vi "GUI_Bella_Control_Center_OFI.vi"() -> ()   [LabVIEW 2020]
uses:
  Shared/GUI_Template/GUI_master/tcp_new_data_event.ctl
  Shared/GUI_Template/GUI_master/tcp new data cluster.ctl
  GUI_TestStand/Fire button.ctl
  Device Drivers/DG645/subVIs/TriggerSource_TypDef.ctl
  Jet on times.ctl
  <vilib>/Utility/config.llb/Write Key (I32).vi
  <vilib>/Platform/browser.llb/Open URL in Default Browser (string).vi
  <vilib>/Utility/config.llb/NI_LVConfig.lvlib
panel:
  out "Jet On Times":T1 {"gas jet on time" format="%#_6p"}
  in  "value10::42":dbl=0.006 caption="JetOnTime H" min=0.0 max=0.01 format="%#_6p"
  in  "value9::42":dbl=0.006 caption="JetOnTime F" min=0.0 max=0.01 format="%#_6p"
  in  "value8::42":dbl=0.006 caption="JetOnTime D" min=0.0 max=0.01 format="%#_6p"
  in  "Delay.Ch H::32":dbl caption="Time width H" min=-0.1 max=0.01 format="%.3p"
  in  "Delay.Ch G::32":dbl caption="jet open G" min=-0.1 max=0.1 format="%.3p"
  in  "Delay.Ch D::32":dbl caption="Time Width D" min=-0.1 max=0.01 format="%.3p"
  in  "Delay.Ch E::32":dbl caption="jet open E" min=-0.1 max=0.03 format="%.3p"
  in  "Delay.Ch F::32":dbl caption="Time width F" min=-0.1 max=0.01 format="%.3p"
  in  "Delay.Ch C::32":dbl caption="jet open C" min=-0.1 max=0.1 format="%.3p"
  out "got manpar ofi bool data":bool
  out "got manpar ofi data":bool
  out "set expt editor":bool
  in  "Delay.Ch B::10":dbl=-1.631e-06 caption="UniblitzOpenTime\n(0 closed, 0.07 default)" min=-0.1 max=0.08 format="%.4f"
  in  "Delay.Ch D::10":dbl=-1.631e-06 caption="Delay D" min=-0.1 max=0.01 format="%.4f"
  in  "value6::42":dbl=0.006 caption="PostScanRate" min=0.1 max=1.0 format="%#_3f"
  in  "value5::42":dbl=0.006 caption="1BL-2BL-\nSplitter-Rpcnt" min=-9999999.0 max=9999999.0 format="%#_6p"
  in  "value6::43":bool=TRUE caption="GhostFoil-In"
  in  "value5::43":bool=TRUE caption="1BL-Energy\nMeter-In"
  in  "value4::43":bool=TRUE caption="2BLFoil-In"
  in  "value3::43":bool=TRUE caption="1BLFoil-In"
  in  "value2::43":bool=TRUE caption="ClunkerIn"
  out "CurrentStatus":string
  in  "MoveStage":bool
  in  "Position.Ch1::44":dbl caption="Current Position" min=0.0 max=150.0
  in  "GUIdevice 44":string="STAGE-LT-Megattenuator"
  in  "GUIdevice 43":string="MANPAR-BELLA-OFI-Boolean"
  in  "GUIdevice 42":string="MANPAR-BELLA-OFI"
  in  "Pressure.device 2::39":dbl caption="Dopant pressure\nLow1down" min=-20.0 max=500.0 format="%.3f"
  out "HPD2 to match HPD":dbl
  in  "Save \ncreenshots":bool
  out "error out":errorcluster
  out "Hpd pos for jet exit":dbl
  in  "value2::42":dbl=276.0 caption="jet exit on hpd for hexX=0" min=-9999999.0 max=9999999.0
  in  "GUIdevice 41":string="STAGE-PL1-JetLength"
  in  "position::41":dbl caption="Jet Length pos" min=0.0 max=50.0 format="%.1f"
  out "lp mode HPDplane\n - HPD ref pos":dbl
  out "height above jet":dbl
  in  "value3::42":dbl=2.6 caption="zpos for 0 above jet" min=-9999999.0 max=9999999.0
  out "HPD - focus":dbl
  in  "value1::42":dbl=230.0 caption="focus on HPD" min=-9999999.0 max=9999999.0
  out "1BL delay (ns)\n+ is 1BL after 2BL":dbl
  in  "Position.Axis 1::8":dbl caption="1BL delay (mm)" min=-500.0 max=500.0 format="%.1f"
  in  "GUIdevice 8":string="STAGE-LT-1BLDelay"
  in  "value4::42":dbl=0.006 caption="JetOnTime B" min=-9999999.0 max=9999999.0 format="%#_6p"
  in  "Position.Channel 5::25":dbl caption="SMFiber (45in, 1out)" min=-60.0 max=55.0 format="%.1f"
  in  "value1::43":bool=TRUE caption="GasJetOn"
  in  "value0::43":bool=TRUE caption="SCS"
  in  "Thales.DIAG_CU_Output_Percent_1::37":dbl caption="Amp2 att (%)" min=1.0 max=100.0 step=500.0 format="%.2f"
  in  "GUIdevice 37":string="SVE-LT-Thales"
  in  "Pressure.device 1::39":dbl caption="Hydrogen pressure\nHigh500" min=-20.0 max=500.0 format="%.3f"
  in  "GUIdevice 39":string="PRC-PL1-HighPressure"
  in  "Scan":T2(ring)
  in  "LogTable":bool
  in  "New Google\nExpLog for new day?":bool=TRUE
  out "standard output":string
  in  "Create Log":bool caption="LogTable"
  in  "GUIdevice 38":string="STAGE-2BL-Compressor"
  in  "Position.Axis 1::38":dbl caption="Comp2 Translation" min=0.0 max=20.0 format="%.3f"
  in  "Position.Channel 5::31":T3(ring) caption="FROG foil"
  in  "Position.Channel 2::31":T3(ring) caption="Little Rick"
  in  "AnalogOutput.Channel 1::36":dbl caption="M4A att (V)" min=0.0 max=5.0 step=500.0 format="%.2f"
  in  "GUIdevice 36":string="ATT-2BL-M4A"
  in  "GUIdevice 35":string="ATT-2BL-DM"
  in  "AnalogOutput.Channel 1::35":dbl caption="2BL DM att (V)" min=0.0 max=5.0 step=500.0 format="%.2f"
  in  "Step size 2":dbl=20.0 caption="Step size" min=-22.0 max=22.0
  in  "Position.Axis 4::33":dbl caption="Holy M V F4" min=-100000.0 max=100000.0 step=500.0
  in  "Position.Axis 3::33":dbl caption="Holy M H F3" min=-1000000.0 max=1000000.0 step=500.0
  in  "Position.Axis 2::33":dbl caption="Bessel M3 V F2" min=-100000.0 max=100000.0 step=500.0
  in  "Position.Axis 1::33":dbl caption="Bessel M3 H F1" min=-100000.0 max=100000.0 step=500.0
  in  "GUIdevice 33":string="MCD-PL1-picosOFI1"
  in  "Delay.Ch B::32":dbl caption="Time width B" min=-0.1 max=0.01 format="%.3p"
  in  "Delay.Ch A::32":dbl caption="jet open A" min=-0.1 max=0.1 format="%.3p"
  in  "GUIdevice 32":string="DDG-AA-SRSGasJet-645"
  in  "position::6":dbl caption="LPmode stage long (605 safe)" min=0.0 max=605.0 format="%.1f"
  in  "GUIdevice 6":string="STAGE-PL1-LPmodeLong"
  in  "EnableMotor::6":bool caption="LPmode motor \nstatus"
  in  "GUIdevice 4":string="STAGE-PL1-Capstage1"
  in  "GUIdevice 31":string="1WIRE-BELLA-Flipper"
  in  "Amplitude.Ch GH::10":dbl=-1.631e-06 caption="Shot Shutter V" min=0.5 max=5.0 format="%.1f"
  in  "Rate (Hz)":dbl=0.3
  out "Crystal2":enum16{"In", "Out", "Unknown"}(ring)
  in  "wangle::28":dbl caption="w" min=-2.0 max=2.0 step=0.01 format="%.5f"
  in  "vangle::28":dbl caption="v" min=-5.0 max=5.0 step=0.01 format="%.5f"
  in  "uangle::28":dbl caption="u" min=-1.0 max=1.0 step=0.01 format="%.5f"
  in  "ypos::28":dbl caption="y" min=-3.0 max=3.0 step=0.01 format="%.5f"
  in  "zpos::28":dbl caption="z" min=-12.5 max=12.5 step=0.01 format="%.5f"
  in  "xpos::28":dbl caption="x" min=-0.5 max=0.5 step=0.01 format="%.5f"
  in  "GUIdevice 28":string="HEX-PL1-2"
  in  "Position.Channel 1::25":dbl caption="LPmode kicker (~1in, 75out)" min=-75.0 max=79.0 format="%.1f"
  in  "GUIdevice 25":string="STAGE-PL1-Smaract"
  in  "Heater Alignment Directions":bool
  in  "Position.Axis 3::15":dbl caption="XY" min=-3.0 max=16.0 format="%.4f"
  in  "Position.Axis 2::15":dbl caption="Y" min=-3.0 max=17.0 format="%.4f"
  in  "Position.Axis 1::15":dbl caption="X" min=-3.0 max=13.0 format="%.4f"
  in  "GUIdevice 24":string="STAGE-HEAT-TL1"
  in  "Encoder position::23":dbl caption="position HPD2" min=0.0 max=600.0 format="%.1f"
  in  "position::3":dbl caption="position HPD" min=0.0 max=600.0 format="%.1f"
  in  "GUIdevice 23":string="STAGE-HPD-Far"
  in  "GUIdevice 22":string="MANPAR-BELLA-FireCont"
  in  "Allow Fire Continues":bool
  out "Fire continues Indicator":bool caption="firing"
  in  "Fire Button":T4=TRUE
  in  "Trigger.Source::10":T5 caption="SRS Trigger Mode"
  out "Absolute discharge timing":dbl caption="delay from pk" format="%#.3p"
  in  "Delay.Ch E::17":dbl caption="Timing box" min=-0.1 max=0.1 format="%.3p"
  in  "value0::22":bool caption="Fire continuosly"
  in  "GUIdevice 15":string="MCD-HEAT-ESP1"
  in  "GUIdevice 17":string="DDG-AA-SRS0"
  out "error IO 2":errorcluster
  out "fire::10":string
  out "tcp data event":T6
  in  "UDP error message":string
  in  "GUIdevice 13":string="DDG-AA-SRS2"
  in  "GUIdevice 2":string="MANPAR-BELLA-General"
  in  "GUIdevice 10":string="DDG-AA-ShotCntrl"
  in  "GUIdevice 1":string="HEX-PL1-1"
  in  "GUIdevice 3":string="STAGE-HPD-Tel"
  in  "<command>::1":bool caption="ABORT\nHEXAPOD"
  in  "Step size":dbl min=-22.0 max=22.0 format="%.5f"
  in  "wangle::1":dbl caption="w (F11 F12)" min=-6.0 max=6.0 step=0.01 format="%.5f"
  in  "vangle::1":dbl caption="v (F9 F10)" min=-6.0 max=1.0 step=0.01 format="%.5f"
  in  "uangle::1":dbl caption="u (F7 F8)" min=-6.0 max=6.0 step=0.01 format="%.5f"
  in  "ypos::1":dbl caption="y (F3 F4)" min=-8.0 max=8.0 step=0.01 format="%.5f"
  in  "zpos::1":dbl caption="z (PgU PgD)" min=-12.0 max=15.0 step=0.01 format="%.5f"
  in  "xpos::1":dbl caption="x (F1 F2)" min=-25.0 max=22.0 step=0.01 format="%.5f"
  in  "Position.Axis 1::9":dbl caption="Comp1 Translation" min=-50.0 max=50.0 format="%.3f"
  in  "GUIdevice 9":string="STAGE-1BL-Compression"
  in  "stop":bool
  # "BELLA CONTROL CENTER"
  # "HEX 1 JET"
  # "HEX 2 Axicon"
  # "Jet"
  # "Discharge timing (s)"
  # "Scan"
  # "1wire"
  # "DG"
  # "\"-x\" is laser propagation direction"
  # "Heater timing (s)"
  # "HPD Stage"
  # "PL1 stages"
  # "Megattenuator Stage"
  # "needs manpar-bella-ofi on\nMANPAR-BELLA-OFI-Boolean"
  # "Attenuate"
  # "OUT"
  # "PICOS"
  # "IN"
  # "Compressors"
  # "Heater Alignment"
  # "Heat ESP0"
  # "Heat ESP1"
  # "Heat Pico"
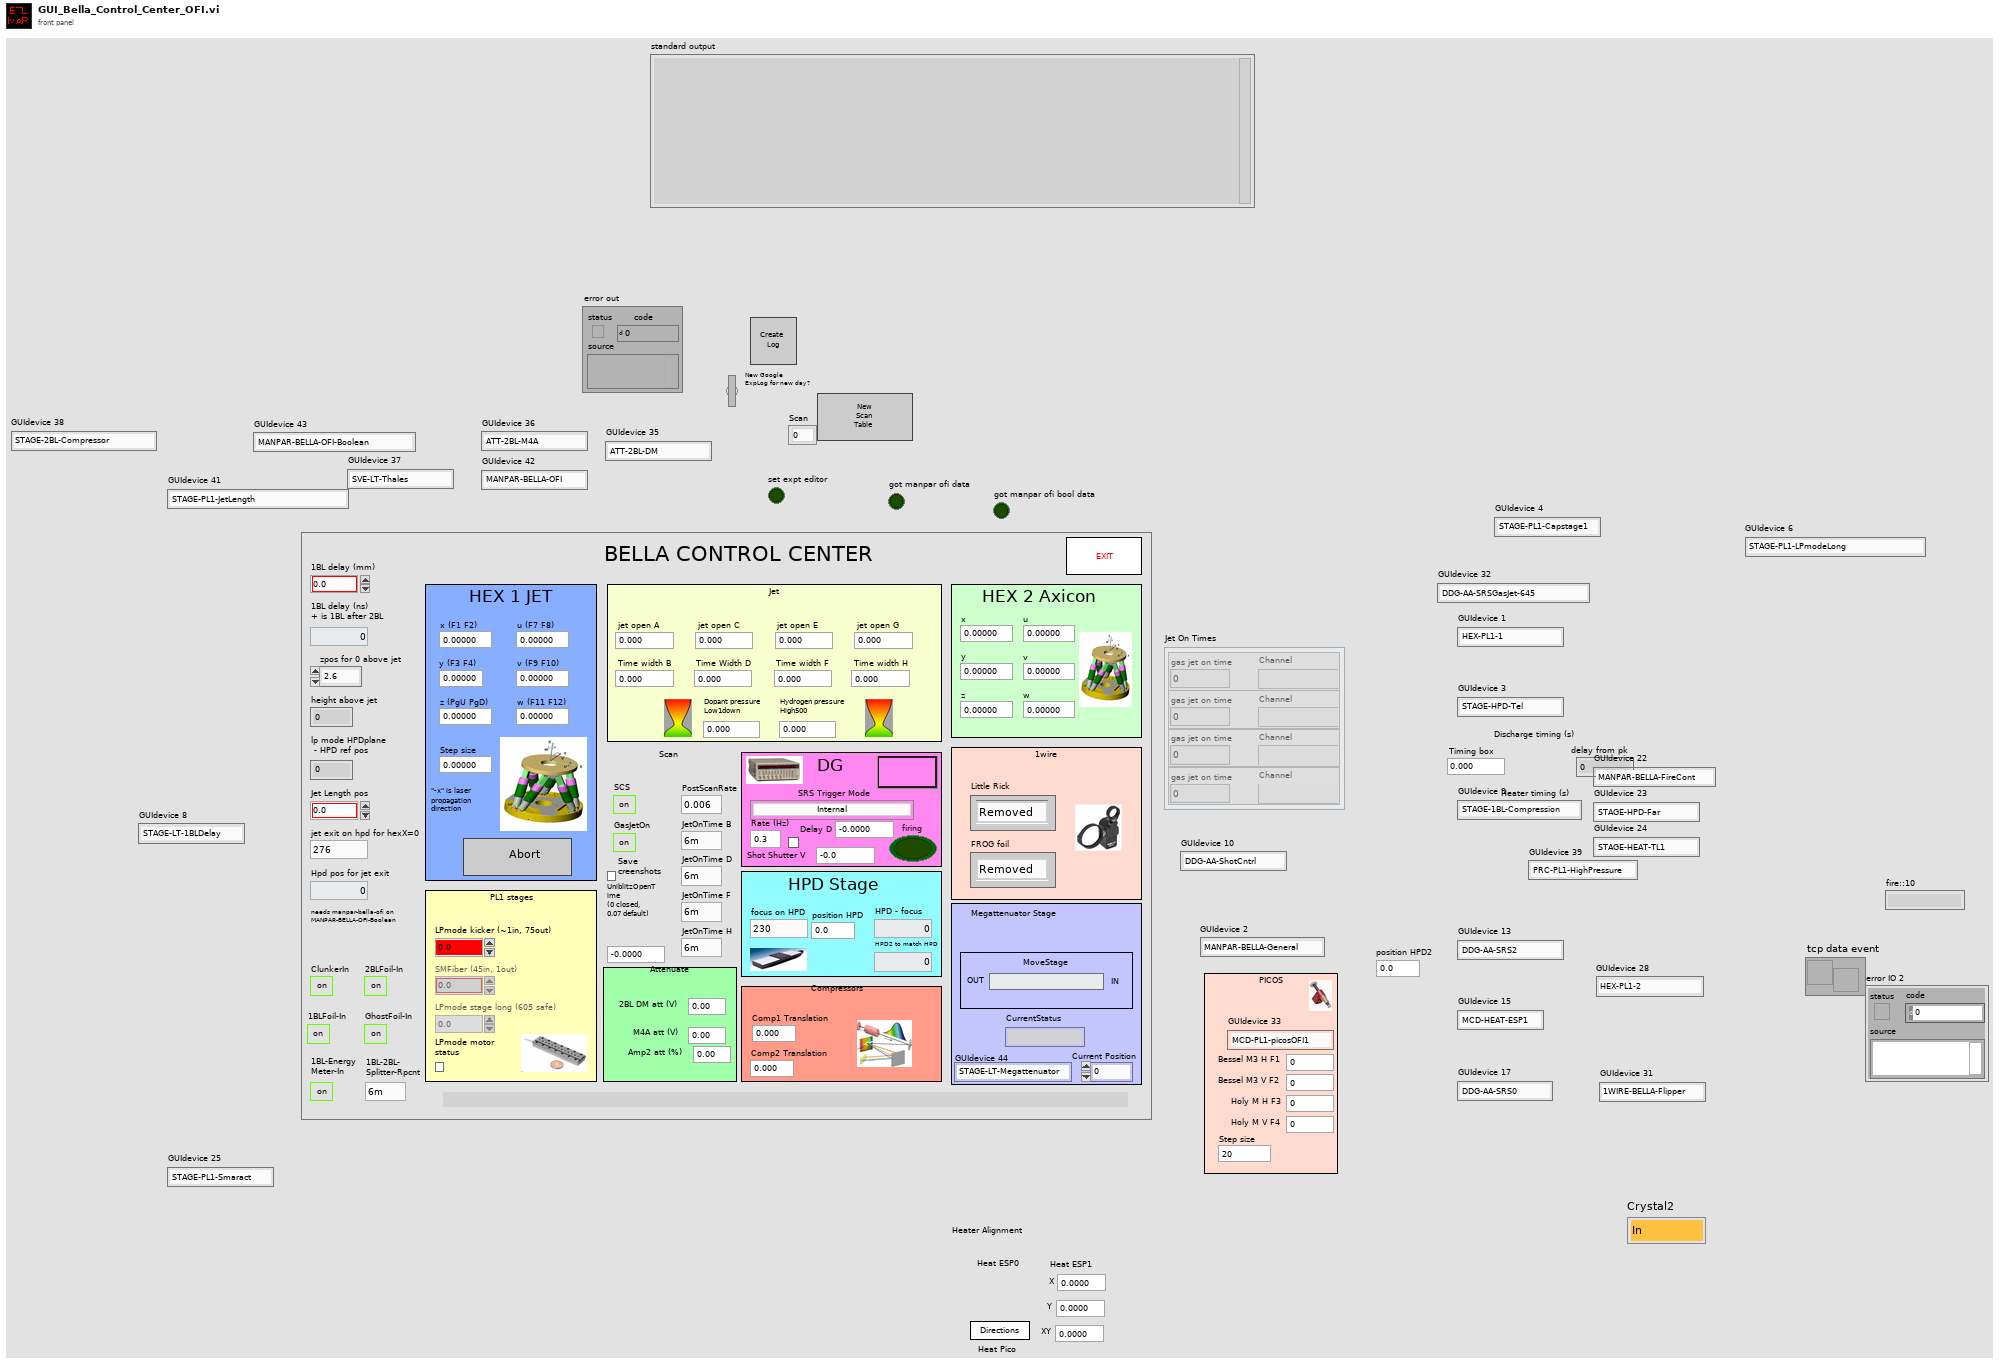
[diagram p1: front panel]
types:
  T1 = typedef "Jet on times.ctl" = cluster{"gas jet on time":dbl, "Channel":string}[]
  T2 = enum16{"0", "1", "2", "3", "4", "5", "6", "7", "8", "9", "10", "11", "12", "13", "14", "15", "16", "17", "18", "19", "20", "21", "22", "23", "24", "25", "26", "27", "28", "29", "30", "31", "32", "33", "34", "35", "36", "37", "38", "39", "40", "41", "42", "43", "44", "45", "46", "47", "48", "49", "50", "51", "52", "53", "54", "55", "56", "57", "58", "59", "60", "61", "62", "63", "64", "65", "66", "67", "68", "69", "70", "71", "72", "73", "74", "75", "76", "77", "78", "79", "81", "82", "83", "84", "85", "86", "87", "88", "89", "90", "91", "92", "93", "94", "95", "96", "97", "98", "99", ""}
  T3 = enum16{"Removed", "Inserted", "Unknown", "Moving"}
  T4 = typedef "Fire button.ctl" = bool
  T5 = typedef "TriggerSource_TypDef.ctl" = enum16{"Internal", "External rising edges", "External falling edges", "Single shot external rising edges", "Single shot external falling edges", "Single shot", "Line"}
  T6 = typedef "tcp_new_data_event.ctl" = refnum<user-event>
  T7 = typedef "tcp new data cluster.ctl" = cluster{"EventEnum":enum16{"new data", "connection status update"}, "Device name":string}
  T8 = enum8{"Enabled", "Disabled", "Disabled and Grayed Out"}
  T9 = enum32{"invalid app kind", "Development System", "Run Time System", "Student Edition", "Embedded LabVIEW", "Evaluation", "Custom"}
  T10 = enum32{"Invalid", "Standard", "Closed", "Hidden", "Minimized", "Maximized"}
  T11 = typedef "imagedata.ctl" = cluster{"image type":i32, "image depth":i32, "image":u8[], "mask":u8[], "colors":u32[], "Rectangle":cluster{"left":i16, "top":i16, "right":i16, "bottom":i16}}
  T12 = typedef "NI_LVConfig.lvlib/Config Data RefNum.ctl" = refnum<k1>
  T13 = cluster{"Core":cluster{"Current VI Reference":refnum<vi>, "Close Panel on Exit?":bool}, "Heater timing offset":dbl, "Discharge timing offset":dbl, "Jet trigger":bool, "Tik1":u32, "Tik2":u32, "Fire Continues Allowed":bool}
  T14 = cluster{"Current VI Reference":refnum<vi>, "Close Panel on Exit?":bool}
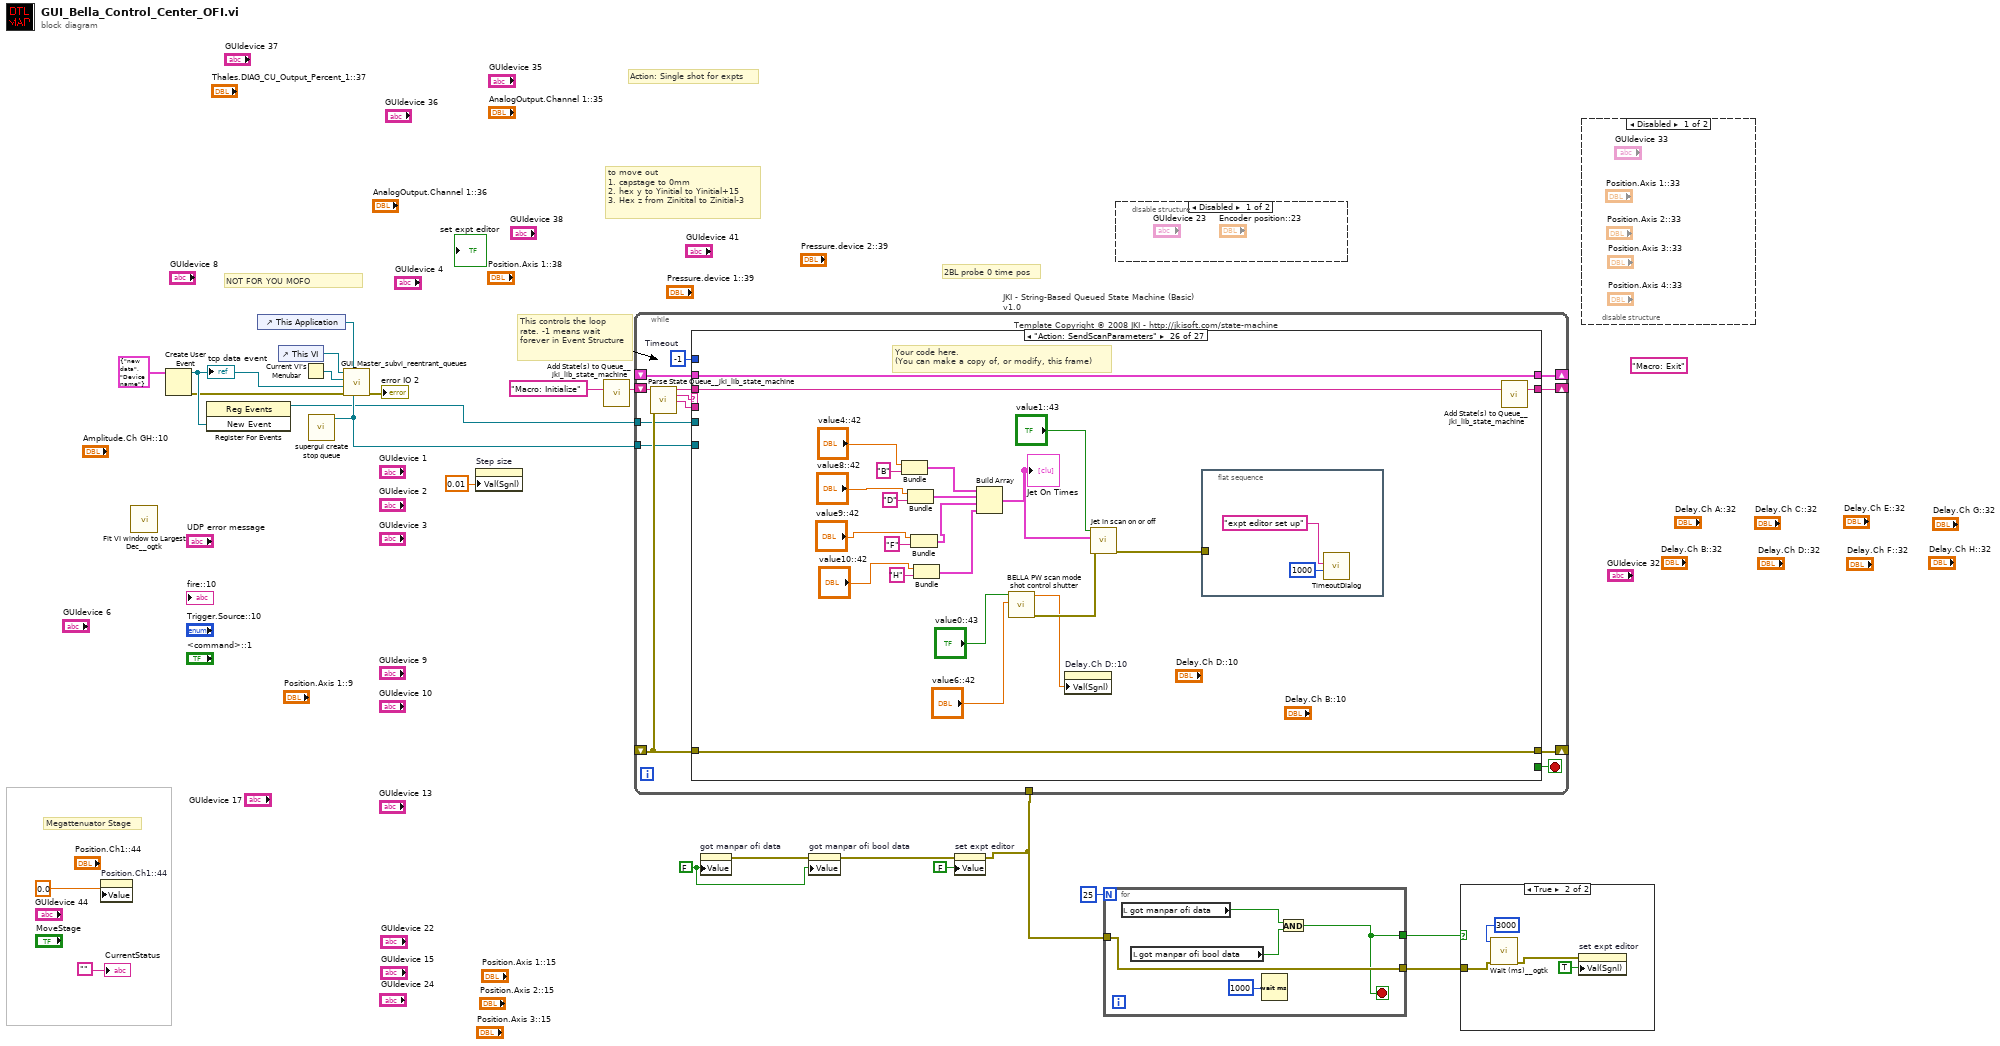
[diagram p0: block diagram]
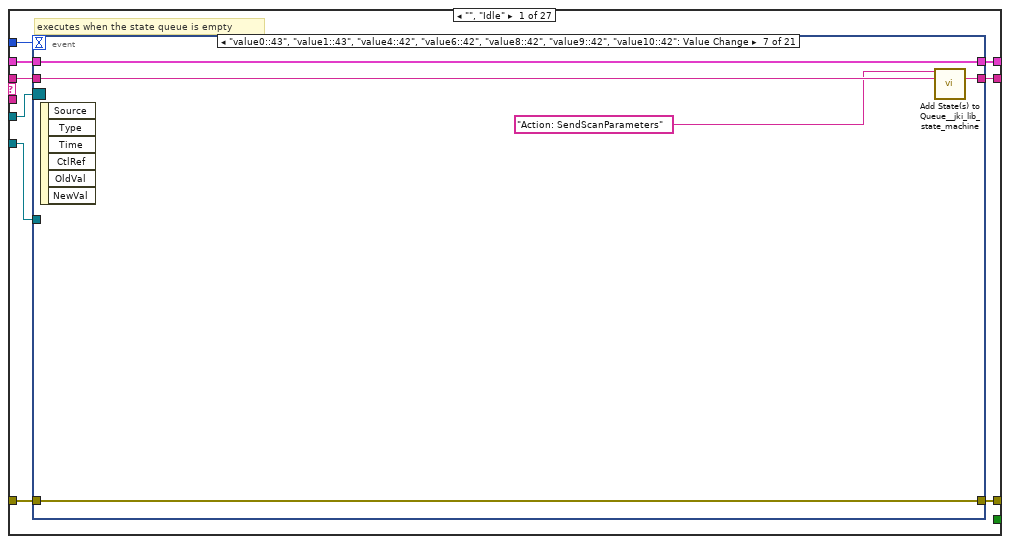
[diagram p5: hidden frame]
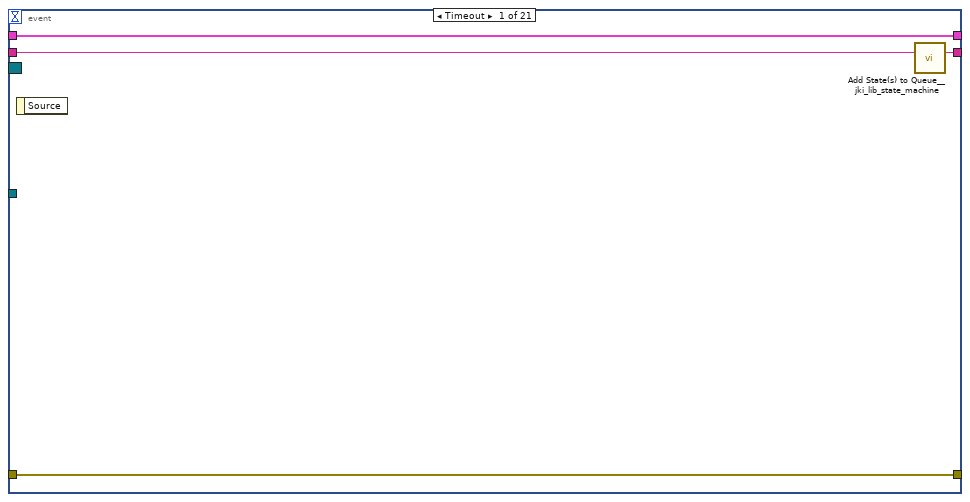
[diagram p6: hidden frame]
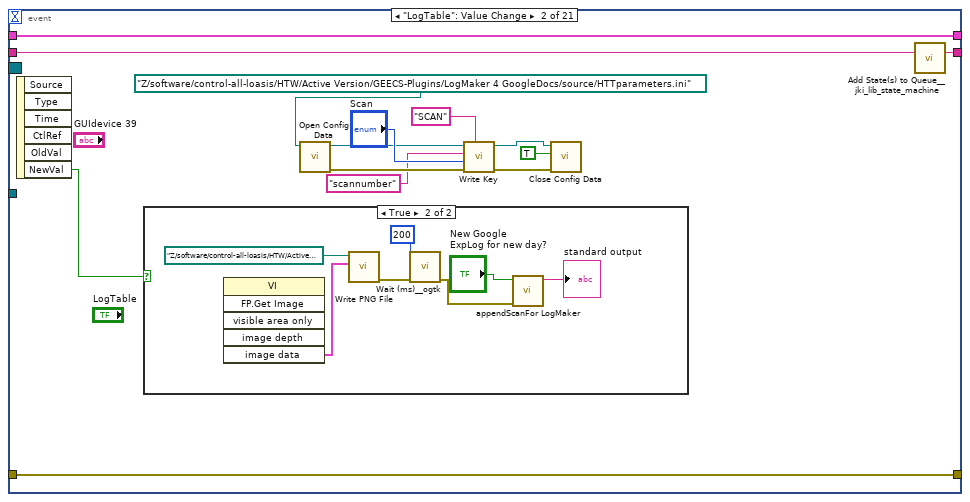
[diagram p7: hidden frame]
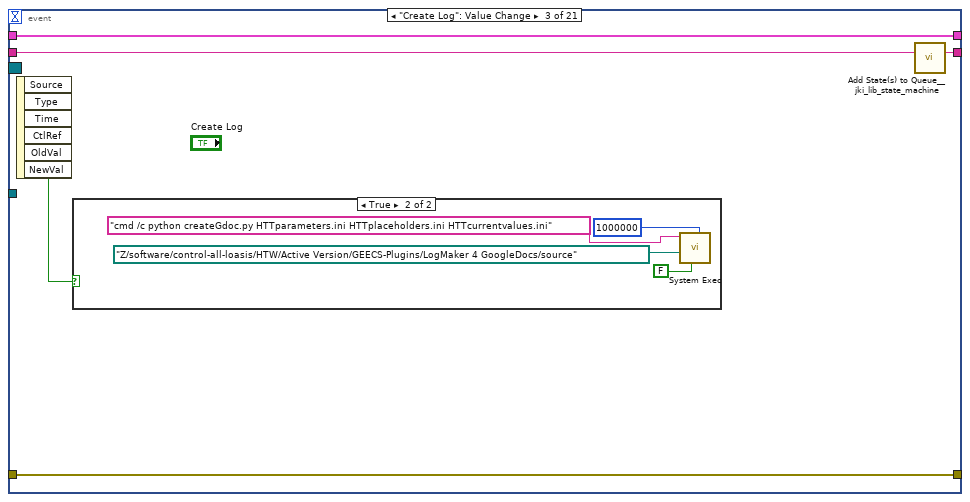
[diagram p9: hidden frame]
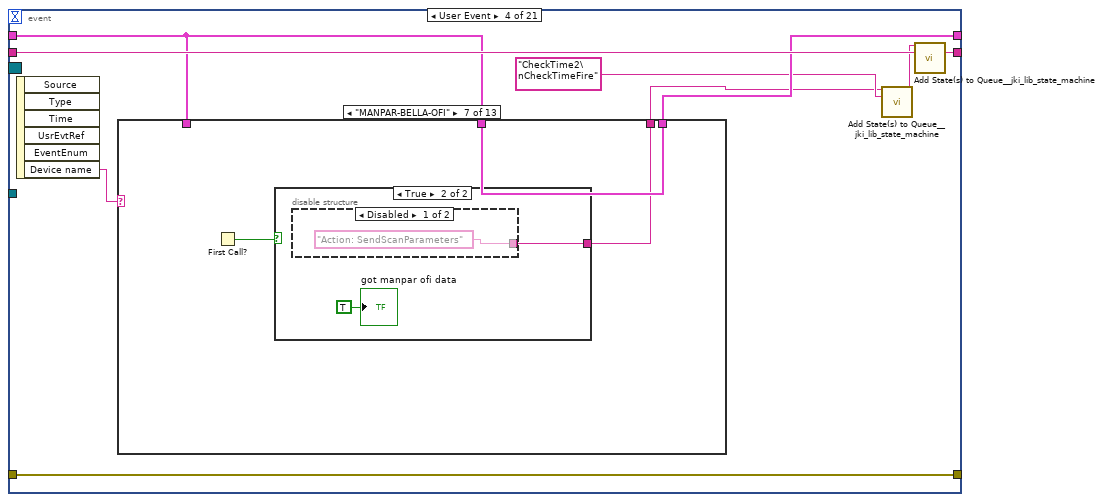
[diagram p11: hidden frame]
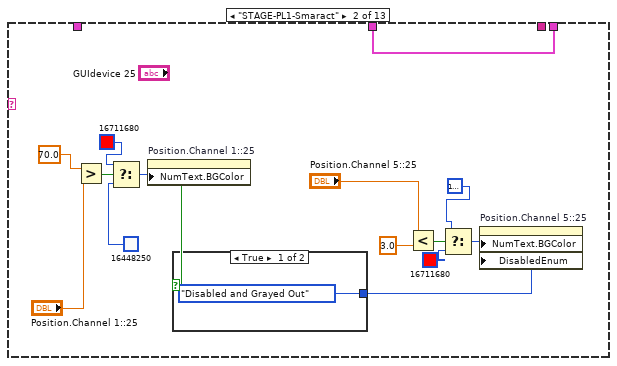
[diagram p13: hidden frame]
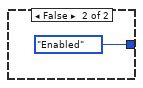
[diagram p14: hidden frame]
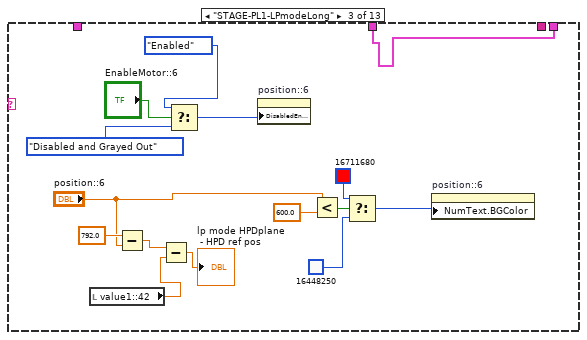
[diagram p15: hidden frame]
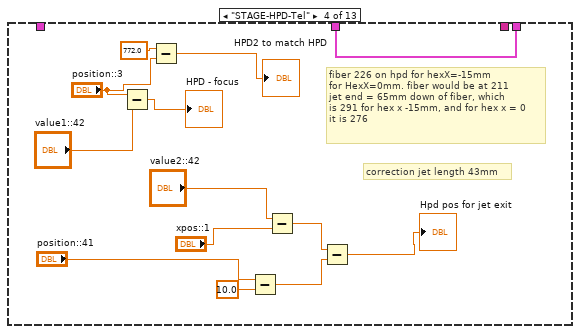
[diagram p16: hidden frame]
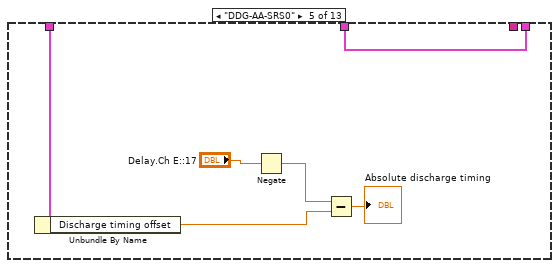
[diagram p17: hidden frame]
diagram:
  w5 = FALSE ("got manpar ofi data")
  (unwired) "Macro: Exit"
  # "Megattenuator Stage"
  # "2BL probe 0 time pos"
  # "Action: Single shot for expts"
  # "to move out\n1. capstage to 0mm\n2. hex y to Yinitial to Yinitial+15\n3. Hex z from Zinitital to Zinitial-3"
  # "This controls the loop rate. -1 means wait forever in Event Structure"
  # "NOT FOR YOU MOFO"
  n1 = property on="Position.Ch1::44" class="DigNum (strict)"("Value"=0.0 ("Position.Ch1::44")) -> ()  [unwired: 2 in, 2 out]
  n2 = call <userlib>:"Fit VI window to Largest Dec__ogtk.vi"() -> ()  [unwired: 6 in, 2 out]
  n3 = Create User Event(user event datatype=T7 {"EventEnum"=enum."new data", "Device name"="Device name"} ("New Event")) -> (user event=w21:refnum<user-event>, error out=w20:errorcluster)  [unwired: 1 in]
  "tcp data event" <- w21
  n4 = register-events(w21) -> (reference out=w11:refnum<event-registration>)  [unwired: 2 in, 1 out]
  n5 = control-ref of="This Application"() -> (w22:refnum<vi>)
  n6 = control-ref of="This VI"() -> (w15:refnum<vi>)
  n7 = Current VI's Menubar() -> (w18:refnum<k9>)
  n8 = call "supergui create stop queue.vi"() -> ("STOP Queue out"=w12:refnum<queue>)  [unwired: 11 in]
  n9 = call "GUI_Master_subvi_reentrant_queues.vi"("STOP Queue in"=w12, "This Application"=w22, "error in (no error)"=w20, "tcp data event"=w21, "Caller menu reference"=w18, "Caller VI ref"=w15) -> ("error out"=→"error IO 2":errorcluster)  [unwired: 5 in]
  n10 = property on="Step size" class="DigNum (strict)"("Val(Sgnl)"=0.01 ("Value (Signaling)")) -> ()  [unwired: 2 in, 2 out]
  n11 = call <vilib>:"Add State(s) to Queue__jki_lib_state_machine.vi"("State(s) in (\"\")"="Macro: Initialize") -> ("States Out"=w13:string)  [unwired: 14 in]
  n12 = property on="got manpar ofi data" class="Bool (strict)"("Value"=w5) -> (error out=w6:errorcluster)  [unwired: 2 in, 1 out]
  n13 = property on="got manpar ofi bool data" class="Bool (strict)"(error in=w6, "Value"=w5) -> (error out=w7:errorcluster)  [unwired: 1 in, 1 out]
  n14 = property on="set expt editor" class="Bool (strict)"(error in=w7, "Value"=FALSE ("set expt editor")) -> (error out=w4:errorcluster)  [unwired: 1 in, 1 out]
  n15 = while "JKI - String-Based Queued State Machine (Basic) v1.0" {
    shift-right: [w28] -> _
    shift-left: _ -> [w27]
    shift-right: [w31] -> _
    shift-left: _ -> [w25]
    shift-right: [w30] -> _
    shift-left: w13 -> [w32]
    tunnel: w11 -> [w24]
    tunnel: w12 -> [w23]
    tunnel: w4 -> [_]
    stop <- w29 stop-if-true
    w26 = -1  # Timeout
    # "Template Copyright © 2008 JKI - http://jkisoft.com/state-machine"
    n16 = call <vilib>:"Parse State Queue__jki_lib_state_machine.vi"("State Queue"=w32, "Error In (no error)"=w25) -> ("Remaining States"=w34:string, "Current State"=w35:string, "Arguments"=w33:string)  [unwired: 11 in]
    n17 = case shown="\"Action: SendScanParameters\"" w35 {
      selector: w35 -> [_ _ w355 _ _ _ _ _ _ _ _ _ _ _ _ _ _ _ _ _ _ _ _ _ _ _ _]
      tunnel: w34 -> [w44 w354 w359 w377 w383 w388 w392 w403 w409 w413 w417 w423 w434 w460 w465 w478 w482 w488 w497 w534 w545 w557 w569 w578 w582 w605 w612]
      tunnel: w33 -> [_ _ _ _ _ _ _ _ _ _ _ w418 w428 _ _ _ _ _ _ _ _ _ _ _ _ _ _]
      tunnel: w27 -> [w42 w351 w357 w368 w380 w386 w389 _ w404 w410 w415 w421 w430 w457 w462 w475 w479 w485 w494 w522 w541 w551 w566 w576 w579 w602 w609]
      tunnel: [w41 w352 w361 w374 errorcluster {"status"=FALSE, "code"=0, "source"=""} ("error out") w385 w390 w400 w405 w411 w414 w419 w431 w458 w463 w476 w480 w486 w495 w532 w539 w546 w567 w573 w580 w603 w610] -> w31
      tunnel: w25 -> [w40 w352 w360 w374 w379 w385 w390 w400 w406 w411 w414 w420 w432 w458 w463 w476 w480 w486 w495 w532 w543 w547 w567 w574 w580 w603 w610]
      tunnel: [w43 w353 w358 w376 w382 w387 w391 w402 w408 w412 w416 w422 w433 w459 w464 w477 w481 w487 w496 w533 w544 w556 w568 w577 w581 w604 w611] -> w30
      tunnel: [_ _ _ _ _ TRUE _ _ _ _ _ _ _ _ _ _ _ _ _ _ _ _ _ _ _ _ _] -> w29
      tunnel: [w36 w351 w357 w375 w380 w386 w389 w401 w404 w410 w415 w421 w430 w457 w462 w475 w479 w485 w494 w531 w541 w550 w565 w576 w579 w602 w609] -> w28
      tunnel: w26 -> [w39 _ _ _ _ _ _ _ _ _ _ _ _ _ _ _ _ _ _ _ _ _ _ _ _ _ _]
      tunnel: w24 -> [w38 _ _ _ _ _ _ _ _ _ _ _ _ _ _ _ _ _ _ _ _ _ _ _ _ _ _]
      tunnel: w23 -> [w37 _ _ _ _ _ _ _ _ _ _ _ _ _ _ w467 _ _ _ _ _ _ _ _ _ _ _]
      frame "", "Idle" {
        # "executes when the state queue is empty"
        n18 = event shown="[6] \"value0::43\", \"value1::43\", \"value4::42\", \"value6::42\", \"value8::42\", \"value9::42\", \"value10::42\": Value Change" {
          selector: w38 -> [_ _ _ _ _ _ _ _ _ _ _ _ _ _ _ _ _ _ _ _ _]
          dyn-events: _ -> [_ _ _ _ _ _ _ _ _ _ _ _ _ _ _ _ _ _ _ _ _]
          timeout: w39 -> [_ _ _ _ _ _ _ _ _ _ _ _ _ _ _ _ _ _ _ _ _]
          tunnel: w44 -> [w48 w62 w74 w87 w194 w196 w201 w211 w221 w231 w241 w251 w260 w268 w277 w300 w305 w315 w322 w324 w350]
          tunnel: [w47 w61 w73 w86 w193 w197 w202 w212 w222 w232 w242 w252 w261 w268 w276 w300 w303 w315 w322 w323 w349] -> w43
          tunnel: w42 -> [w45 w59 w71 w83 w191 w199 w204 w214 w224 w234 w244 w254 w263 w267 w279 w301 w307 w316 w321 w331 w347]
          tunnel: [w46 w60 w72 w85 w192 w198 w203 w213 w223 w233 w243 w253 w262 w265 w282 w299 w306 w314 w320 w330 w348] -> w41
          tunnel: w40 -> [w46 w60 w72 w85 w192 w198 w203 w213 w223 w233 w243 w253 w262 w266 w281 w299 w306 w314 w320 w330 w348]
          tunnel: [w45 w59 w71 w82 w191 w199 w204 w214 w224 w234 w244 w254 w263 w267 w280 w301 w307 w316 w321 w331 w347] -> w36
          tunnel: w37 -> [_ _ _ _ _ _ _ _ _ _ _ _ _ _ _ _ _ _ _ _ _]
          event Timeout {
            n19 = event-data() -> ()  [unwired: 1 in, 1 out]
            n20 = call <vilib>:"Add State(s) to Queue__jki_lib_state_machine.vi"("State(s) in (\"\")"=w48) -> ("States Out"=w47:string)  [unwired: 14 in]
          }
          event "LogTable": Value Change {
            n21 = event-data() -> ("NewVal"=w49:bool)  [unwired: 1 in, 5 out]
            n22 = case shown="True" w49 {
              frame False {
              }
              frame True {
                n23 = invoke class="VI" method="FP.Get Image"() -> ("image data"=w69:T11)  [unwired: 6 in, 5 out]
                n24 = call <vilib>:"Write PNG File.vi"("image data"=w69, "path to PNG file"=path "Z:/software/control-all-loasis/HTW/Active Version/GEECS-Plugins/LogMaker 4 GoogleDocs/source/frontpanel.png" ("report file path")) -> ("error out"=w64:errorcluster)  [unwired: 8 in, 1 out]
                n25 = call <userlib>:"Wait (ms)__ogtk.vi"("error in (no error)"=w64, "milliseconds to wait"=u32 200 ("millisecond timer value")) -> ("error out"=w63:errorcluster)  [unwired: 8 in, 1 out]
                n26 = call "appendScanFor LogMaker.vi"("error in (no error)"=w63, "New Google\nExpLog for new day?"="New Google\nExpLog for new day?") -> ("standard output"=→"standard output":string)  [unwired: 9 in]
              }
            }
            n27 = call <vilib>:"Open Config Data.vi"("configuration file path"=path "Z:/software/control-all-loasis/HTW/Active Version/GEECS-Plugins/LogMaker 4 GoogleDocs/source/HTTparameters.ini") -> ("error out"=w56:errorcluster, "refnum"=w54:T12)  [unwired: 8 in, 1 out]
            n28 = call-poly <vilib>:"Write Key.vi"("section"="SCAN", "error in (no error)"=w56, "value"="Scan", "key"="scannumber", "refnum"=w54) -> ("error out"=w57:errorcluster, "refnum out"=w55:T12)  [unwired: 4 in, 1 out]
            n29 = call <vilib>:"Close Config Data.vi"("error in (no error)"=w57, "write file if changed (T)"=TRUE, "refnum"=w55) -> ()  [unwired: 7 in, 2 out]
            n30 = call <vilib>:"Add State(s) to Queue__jki_lib_state_machine.vi"("State(s) in (\"\")"=w62) -> ("States Out"=w61:string)  [unwired: 14 in]
          }
          event "Create Log": Value Change {
            n31 = event-data() -> ("NewVal"=w70:bool)  [unwired: 1 in, 5 out]
            n32 = case shown="True" w70 {
              frame False {
              }
              frame True {
                n33 = call <vilib>:"System Exec.vi"("expected output size  (4096)"=u32 1000000, "run minimized? (F)"=FALSE, "working directory"=path "Z:/software/control-all-loasis/HTW/Active Version/GEECS-Plugins/LogMaker 4 GoogleDocs/source", "command line"="cmd /c python createGdoc.py HTTparameters.ini HTTplaceholders.ini HTTcurrentvalues.ini") -> ()  [unwired: 4 in, 4 out]
              }
            }
            n34 = call <vilib>:"Add State(s) to Queue__jki_lib_state_machine.vi"("State(s) in (\"\")"=w74) -> ("States Out"=w73:string)  [unwired: 14 in]
          }
          event User Event {
            n35 = event-data() -> ("Device name"=w84:string)  [unwired: 1 in, 5 out]
            n36 = case shown="\"MANPAR-BELLA-OFI\"" w84 {
              tunnel: w83 -> [_ _ _ _ w135 _ _ _ _ _ _ _ _]
              tunnel: w83 -> [w88 w102 w119 w132 w133 w139 w142 w148 w155 w160 w167 w169 w189]
              tunnel: [w88 w102 w119 w132 w133 w139 w142 w148 w155 w160 w167 w169 w189] -> w82
              tunnel: [_ _ _ _ _ _ w141 w147 "Check Megattenuator Stage Status" ("State(s) in Front (\"\")") _ _ _ _] -> w79
              frame "False", Default {
              }
              frame "STAGE-PL1-Smaract" {
                n37 = Greater?(x=70.0 ("y"), y="Position.Channel 1::25") -> (0:w89:bool)
                n38 = Select(t=u32 16711680, s=w89, f=u32 16448250) -> (s? t:f=w99:u32)
                n39 = property on="Position.Channel 1::25" class="DigNum (strict)"("NumText.BGColor"=w99) -> ()  [unwired: 2 in, 2 out]
                n40 = case shown="True" w89 {
                  tunnel: [T8."Disabled and Grayed Out" ("Disabled") T8."Enabled" ("Disabled")] -> w90
                  frame True {
                  }
                  frame False {
                  }
                }
                n41 = Less?(x="Position.Channel 5::25", y=3.0) -> (x < y?=w95:bool)
                n42 = Select(t=u32 16777225, s=w95, f=u32 16711680) -> (s? t:f=w98:u32)
                n43 = property on="Position.Channel 5::25" class="DigNum (strict)"("NumText.BGColor"=w98, "DisabledEnum"=w90) -> ()  [unwired: 2 in, 2 out]
              }
              frame "STAGE-PL1-LPmodeLong" {
                n44 = local read "value1::42"() -> (w106:dbl)
                n45 = Subtract(x=792.0, y="position::6") -> (x-y=w107:dbl)
                n46 = Subtract(x=w107, y=w106) -> (x-y=→"lp mode HPDplane\n - HPD ref pos":dbl)
                n47 = Select(t=T8."Enabled" ("Disabled"), s="EnableMotor::6", f=T8."Disabled and Grayed Out" ("Disabled")) -> (s? t:f=w110:T8)
                n48 = property on="position::6" class="DigNum (strict)"("DisabledEnum"=w110) -> ()  [unwired: 2 in, 2 out]
                n49 = Less?(x="position::6", y=600.0) -> (x < y?=w118:bool)
                n50 = Select(t=u32 16711680, s=w118, f=u32 16448250) -> (s? t:f=w114:u32)
                n51 = property on="position::6" class="DigNum (strict)"("NumText.BGColor"=w114) -> ()  [unwired: 2 in, 2 out]
              }
              frame "STAGE-HPD-Tel" {
                # "correction jet length 43mm"
                # "fiber 226 on hpd for hexX=-15mm\nfor HexX=0mm. fiber would be at 211\njet end = 65mm down of fiber, which\nis 291 for hex x -15mm, and for hex x = 0\nit is 276"
                n52 = Subtract(x="position::3", y="value1::42") -> (x-y=→"HPD - focus":dbl)
                n53 = Subtract(x=772.0 ("y"), y="position::3") -> (x-y=→"HPD2 to match HPD":dbl)
                n54 = Subtract(x="position::41", y=10.0) -> (x-y=w124:dbl)
                n55 = Subtract(x="value2::42", y="xpos::1") -> (x-y=w125:dbl)
                n56 = Subtract(x=w125, y=w124) -> (x-y=→"Hpd pos for jet exit":dbl)
              }
              frame "DDG-AA-SRS0" {
                n57 = Unbundle By Name(w135) -> ("Discharge timing offset"=w134:dbl)
                n58 = Negate(x="Delay.Ch E::17") -> (-x=w136:dbl)
                n59 = Subtract(x=w136, y=w134) -> (x-y=→"Absolute discharge timing":dbl)
              }
              frame "STAGE-2BL-ProbeDelay" {
              }
              frame "MANPAR-BELLA-OFI" {
                n60 = First Call?() -> (First Call?: T/F=w140:bool)
                n61 = case shown="True" w140 {
                  tunnel: [_ w144] -> w141
                  frame False {
                  }
                  frame True {
                    n62 = disable-structure shown="Disabled" {
                      disable-tunnel: ["Action: SendScanParameters" ("State(s) in Front (\"\")") _] -> w144
                      frame Disabled {
                      }
                      frame Enabled {
                      }
                    }
                    "got manpar ofi data" <- TRUE ("got manpar ofi data")
                  }
                }
              }
              frame "MANPAR-BELLA-OFI-Boolean" {
                n63 = First Call?() -> (First Call?: T/F=w146:bool)
                n64 = case shown="True" w146 {
                  tunnel: [_ w150] -> w147
                  frame False {
                  }
                  frame True {
                    n65 = disable-structure shown="Disabled" {
                      disable-tunnel: ["Action: SendScanParameters" ("State(s) in Front (\"\")") _] -> w150
                      frame Disabled {
                      }
                      frame Enabled {
                      }
                    }
                    "got manpar ofi bool data" <- TRUE ("got manpar ofi bool data")
                  }
                }
              }
              frame "STAGE-LT-Megattenuator" {
                n66 = property on="Position.Ch1::44" class="DigNum (strict)"() -> ("Caption.FontStrike"=w152:bool)  [unwired: 2 in, 2 out]
                n67 = Not(x=w152) -> (.not. x?=w153:bool)
                n68 = property on="MoveStage" class="Bool (strict)"("Visible"=w153) -> ()  [unwired: 2 in, 2 out]
                n69 = property on="CurrentStatus" class="Str"("Visible"=w153) -> ()  [unwired: 2 in, 2 out]
              }
              frame "STAGE-LT-1BLDelay" {
                n70 = Subtract(x="Position.Axis 1::8", y=929.0) -> (x-y=w165:dbl)
                n71 = Negate(x=w165) -> (-x=w164:dbl)
                n72 = Multiply(x=2.0, y=w164) -> (x*y=w162:dbl)
                n73 = Divide(x=w162, y=299792458000.0) -> (x/y=w159:dbl)
                n74 = Multiply(x=1000000000.0, y=w159) -> (x*y=→"1BL delay (ns)\n+ is 1BL after 2BL":dbl)
              }
              frame "1WIRE-BELLA-Flipper" {
              }
              frame "HEX-PL1-2" {
                n75 = disable-structure shown="Disabled" {
                  disable-tunnel: "ypos::28" -> [w173 _]
                  frame Disabled {
                    n76 = Equal?(x=w173, y=15.6) -> (x = y?=w171:bool)
                    n77 = Equal?(x=-20.0 ("y"), y=w173) -> (x = y?=w175:bool)
                    n78 = case shown="False" w175 {
                      tunnel: [w179 enum16{"In", "Out"}."Out" ("sdfsdfs 2")] -> w170
                      tunnel: [w177 u32 16185078] -> w174
                      tunnel: w171 -> [w178 _]
                      frame False {
                        n79 = case shown="False" w178 {
                          tunnel: [enum16{"In", "Out", "Unknown"}."Unknown" ("sdfsdfs 2") enum16{"In", "Out"}."In" ("sdfsdfs 2")] -> w179
                          tunnel: [u32 16761154 ("Color Box") u32 16711680] -> w177
                          frame False {
                          }
                          frame True {
                          }
                        }
                      }
                      frame True {
                      }
                    }
                    "Crystal2" <- w170
                    n80 = property on="Crystal2" class="Enum (strict)"("RingText.FG Color"=w174, "RingText.BGColor"=w174) -> ()  [unwired: 2 in, 2 out]
                  }
                  frame Enabled {
                  }
                }
              }
              frame "HEX-PL1-1" {
                n81 = Subtract(x="value3::42", y="zpos::1") -> (x-y=→"height above jet":dbl)
              }
            }
            n82 = call <vilib>:"Add State(s) to Queue__jki_lib_state_machine.vi"("State(s) in Front (\"\")"=w79, "State(s) in (\"\")"="CheckTime2\nCheckTimeFire" ("State(s) in Front (\"\")")) -> ("States Out"=w80:string)  [unwired: 13 in]
            n83 = call <vilib>:"Add State(s) to Queue__jki_lib_state_machine.vi"("State(s) in Front (\"\")"=w80, "State(s) in (\"\")"=w87) -> ("States Out"=w86:string)  [unwired: 13 in]
          }
          event "stop": Value Change {
            # "Exit Button Value Change (pressed) Event\n(this executes Macro: Exit to terminate the VI)"
            n84 = event-data() -> ()  [unwired: 1 in, 6 out]
            n85 = call <vilib>:"Add State(s) to Queue__jki_lib_state_machine.vi"("State(s) in Front (\"\")"="Macro: Exit", "State(s) in (\"\")"=w194) -> ("States Out"=w193:string)  [unwired: 13 in]
          }
          event Value Change {
            n86 = event-data() -> ()  [unwired: 1 in, 6 out]
            n87 = call <vilib>:"Add State(s) to Queue__jki_lib_state_machine.vi"("State(s) in Front (\"\")"="Action: Fire" ("State(s) in Front (\"\")"), "State(s) in (\"\")"=w196) -> ("States Out"=w197:string)  [unwired: 13 in]
          }
          event "value0::43", "value1::43", "value4::42", "value6::42", "value8::42", "value9::42", "value10::42": Value Change {
            n88 = event-data() -> ()  [unwired: 1 in, 6 out]
            n89 = call <vilib>:"Add State(s) to Queue__jki_lib_state_machine.vi"("State(s) in Front (\"\")"="Action: SendScanParameters" ("State(s) in Front (\"\")"), "State(s) in (\"\")"=w201) -> ("States Out"=w202:string)  [unwired: 13 in]
          }
          event "value2::43": Value Change {
            n90 = event-data() -> ()  [unwired: 1 in, 6 out]
            n91 = local read "GUIdevice 43"() -> (w205:string)
            n92 = Select(t="on", s="value2::43", f="off") -> (s? t:f=w210:string)
            n93 = call "DefaultValue_Variable_MC.vi"("Variable In"="value2", "Default Value"=w210, "Device In"=w205) -> ()  [unwired: 1 in]
            n94 = call <vilib>:"Add State(s) to Queue__jki_lib_state_machine.vi"("State(s) in (\"\")"=w211) -> ("States Out"=w212:string)  [unwired: 14 in]
          }
          event "value3::43": Value Change {
            n95 = event-data() -> ()  [unwired: 1 in, 6 out]
            n96 = local read "GUIdevice 43"() -> (w216:string)
            n97 = Select(t="on", s="value3::43", f="off") -> (s? t:f=w220:string)
            n98 = call "DefaultValue_Variable_MC.vi"("Variable In"="value3", "Default Value"=w220, "Device In"=w216) -> ()  [unwired: 1 in]
            n99 = call <vilib>:"Add State(s) to Queue__jki_lib_state_machine.vi"("State(s) in (\"\")"=w221) -> ("States Out"=w222:string)  [unwired: 14 in]
          }
          event "value4::43": Value Change {
            n100 = event-data() -> ()  [unwired: 1 in, 6 out]
            n101 = local read "GUIdevice 43"() -> (w226:string)
            n102 = Select(t="on", s="value4::43", f="off") -> (s? t:f=w230:string)
            n103 = call "DefaultValue_Variable_MC.vi"("Variable In"="value4", "Default Value"=w230, "Device In"=w226) -> ()  [unwired: 1 in]
            n104 = call <vilib>:"Add State(s) to Queue__jki_lib_state_machine.vi"("State(s) in (\"\")"=w231) -> ("States Out"=w232:string)  [unwired: 14 in]
          }
          event "value5::43": Value Change {
            n105 = event-data() -> ()  [unwired: 1 in, 6 out]
            n106 = local read "GUIdevice 43"() -> (w236:string)
            n107 = Select(t="on", s="value5::43", f="off") -> (s? t:f=w240:string)
            n108 = call "DefaultValue_Variable_MC.vi"("Variable In"="value5", "Default Value"=w240, "Device In"=w236) -> ()  [unwired: 1 in]
            n109 = call <vilib>:"Add State(s) to Queue__jki_lib_state_machine.vi"("State(s) in (\"\")"=w241) -> ("States Out"=w242:string)  [unwired: 14 in]
          }
          event "value6::43": Value Change {
            n110 = event-data() -> ()  [unwired: 1 in, 6 out]
            n111 = local read "GUIdevice 43"() -> (w246:string)
            n112 = Select(t="on", s="value6::43", f="off") -> (s? t:f=w250:string)
            n113 = call "DefaultValue_Variable_MC.vi"("Variable In"="value6", "Default Value"=w250, "Device In"=w246) -> ()  [unwired: 1 in]
            n114 = call <vilib>:"Add State(s) to Queue__jki_lib_state_machine.vi"("State(s) in (\"\")"=w251) -> ("States Out"=w252:string)  [unwired: 14 in]
          }
          event "value5::42": Value Change {
            n115 = event-data() -> ()  [unwired: 1 in, 6 out]
            n116 = Number To Fractional String(number="value5::42", precision (6)=i16 4) -> (F-format string=w256:string)  [unwired: 2 in]
            n117 = call "DefaultValue_Variable_MC.vi"("Variable In"="value5", "Default Value"=w256, "Device In"="GUIdevice 42") -> ()  [unwired: 1 in]
            n118 = call <vilib>:"Add State(s) to Queue__jki_lib_state_machine.vi"("State(s) in (\"\")"=w260) -> ("States Out"=w261:string)  [unwired: 14 in]
          }
          event "Heater Alignment Directions": Value Change {
            n119 = event-data() -> ()  [unwired: 1 in, 6 out]
            n120 = case shown="True" "Heater Alignment Directions" {
              tunnel: w266 -> [w269 w272]
              tunnel: [w269 w271] -> w265
              frame False {
              }
              frame True {
                n121 = call-poly <vilib>:"Open URL in Default Browser.vi"("error in (no error)"=w272, "URL"="https://docs.google.com/document/d/1RMZp6W8Kkog2nkTymSjyZ2bh9D7Vo4bxhvGgn3Ut4KE/edit") -> ("error out"=w271:errorcluster)  [unwired: 4 in, 1 out]
              }
            }
          }
          event "Allow Fire Continues": Value Change {
            n122 = event-data() -> ()  [unwired: 1 in, 6 out]
            n123 = Unbundle By Name(w279) -> ("Fire Continues Allowed"=w278:bool)
            n124 = case shown="True" "Allow Fire Continues" {
              tunnel: [w283 w290] -> w282
              tunnel: "Allow Fire Continues" -> [_ w289]
              tunnel: w281 -> [w283 w288]
              tunnel: w278 -> [w284 w287]
              tunnel: [w284 w285] -> w274
              tunnel: [_ "Initilize Fire Continues" ("State(s) in Front (\"\")")] -> w273
              frame False {
              }
              frame True {
                n125 = case shown="False" w287 {
                  tunnel: [w296 w297] -> w290
                  tunnel: w289 -> [w295 _]
                  tunnel: w288 -> [w294 w297]
                  tunnel: [w291 FALSE] -> w285
                  frame False {
                    n126 = call "Password"("Enable"=w295, "error in (no error)"=w294) -> ("Password"=w293:string, "error out"=w296:errorcluster)  [unwired: 15 in, 1 out]
                    n127 = Equal?(x=w293, y="fire") -> (x = y?=w291:bool)
                  }
                  frame True {
                  }
                }
              }
            }
            n128 = Bundle By Name(cluster=w279, "Fire Continues Allowed"=w274) -> (w280:T13)
            n129 = call <vilib>:"Add State(s) to Queue__jki_lib_state_machine.vi"("State(s) in Front (\"\")"=w273, "State(s) in (\"\")"=w277) -> ("States Out"=w276:string)  [unwired: 13 in]
          }
          event "Step size": Value Change {
            n130 = event-data() -> ("NewVal"=w302:dbl)  [unwired: 1 in, 5 out]
            n131 = property on="uangle::1" class="DigNum (strict)"("Increment"=w302) -> ()  [unwired: 2 in, 2 out]
            n132 = property on="vangle::1" class="DigNum (strict)"("Increment"=w302) -> ()  [unwired: 2 in, 2 out]
            n133 = property on="xpos::1" class="DigNum (strict)"("Increment"=w302) -> ()  [unwired: 2 in, 2 out]
            n134 = property on="zpos::1" class="DigNum (strict)"("Increment"=w302) -> ()  [unwired: 2 in, 2 out]
            n135 = property on="wangle::1" class="DigNum (strict)"("Increment"=w302) -> ()  [unwired: 2 in, 2 out]
            n136 = property on="ypos::1" class="DigNum (strict)"("Increment"=w302) -> ()  [unwired: 2 in, 2 out]
          }
          event "set expt editor": Value Change {
            n137 = event-data() -> ()  [unwired: 1 in, 6 out]
            n138 = call <vilib>:"Add State(s) to Queue__jki_lib_state_machine.vi"("State(s) in Front (\"\")"="Action: SendScanParameters" ("State(s) in Front (\"\")"), "State(s) in (\"\")"=w305) -> ("States Out"=w303:string)  [unwired: 13 in]
          }
          event "Step size 2": Value Change {
            n139 = event-data() -> ("NewVal"=w308:dbl)  [unwired: 1 in, 5 out]
            n140 = control-ref of="Position.Axis 1::33"() -> (w313:refnum<vi>)
            n141 = control-ref of="Position.Axis 2::33"() -> (w312:refnum<vi>)
            n142 = control-ref of="Position.Axis 4::33"() -> (w310:refnum<vi>)
            n143 = control-ref of="Position.Axis 3::33"() -> (w311:refnum<vi>)
            n144 = Build Array(w313, w312, w311, w310) -> (w309:refnum<vi>[])
            n145 = for {
              tunnel: w309 -> [w318] mode=indexing
              tunnel: w308 -> [w317]
              n146 = property on="Property Node" class="DigNum (strict)"(reference=w318, "Increment"=w317) -> ()  [unwired: 1 in, 2 out]
            }
          }
          event Value Change {
            n147 = event-data() -> ()  [unwired: 1 in, 6 out]
            n148 = property on="value0::22" class="Bool (strict)"("Val(Sgnl)"=FALSE) -> ()  [unwired: 2 in, 2 out]
          }
          event "MoveStage": Value Change {
            n149 = event-data() -> ("OldVal"=w326:bool, "NewVal"=w329:bool)  [unwired: 1 in, 4 out]
            n150 = flat-sequence {
              tunnel: w329 -> [w336]
              tunnel: [w336] -> w328
              tunnel: [w333] -> w327
              tunnel: w326 -> [w332]
              tunnel: [w332] -> w325
              tunnel: w328 -> [w339]
              tunnel: w327 -> [w338]
              tunnel: w325 -> [w337]
              frame #0 {
                n151 = call "PasswordPrompt.vi"() -> ("Please enter password below 2"=w335:string)  [unwired: 11 in]
                n152 = Equal?(x=w335, y="l0dat&srv!") -> (x = y?=w333:bool)
              }
              frame #1 {
                n153 = case shown="True" w338 {
                  tunnel: w339 -> [_ w342]
                  tunnel: w337 -> [w340 _]
                  frame False {
                    n154 = call "Display Message to User"("Message"="Wrong Password") -> ()  [unwired: 9 in, 2 out]
                    n155 = property on="MoveStage" class="Bool (strict)"("Value"=w340) -> ()  [unwired: 2 in, 2 out]
                  }
                  frame True {
                    n156 = case shown="True" w342 {
                      frame False {
                        n157 = property on="Position.Ch1::44" class="DigNum (strict)"("Val(Sgnl)"=150.0 ("Value (Signaling)")) -> ()  [unwired: 2 in, 2 out]
                      }
                      frame True {
                        n158 = property on="Position.Ch1::44" class="DigNum (strict)"("Val(Sgnl)"=0.5 ("Value (Signaling)")) -> ()  [unwired: 2 in, 2 out]
                      }
                    }
                    n159 = property on="MoveStage" class="Bool (strict)"("Value"=w342) -> ()  [unwired: 2 in, 2 out]
                  }
                }
              }
            }
            n160 = call <vilib>:"Add State(s) to Queue__jki_lib_state_machine.vi"("State(s) in (\"\")"=w324) -> ("States Out"=w323:string)  [unwired: 14 in]
          }
          event Panel Close? {
            # "Discard the event because we'll close the front panel ourselves in Macro: Exit"
            # "Close Panel button (pressed) Event\n(this executes Macro: Exit to terminate the VI)"
            n161 = event-data() -> ()  [unwired: 1 in, 1 out]
            n162 = event-data("Discard?"=TRUE) -> ()  [unwired: 1 in, 1 out]
            n163 = call <vilib>:"Add State(s) to Queue__jki_lib_state_machine.vi"("State(s) in Front (\"\")"="Macro: Exit", "State(s) in (\"\")"=w350) -> ("States Out"=w349:string)  [unwired: 13 in]
          }
        }
      }
      frame "---------- Core ----------" {
        # "Do not put any code in this frame.\n(it is a separator no-op)"
        n164 = call <vilib>:"Add State(s) to Queue__jki_lib_state_machine.vi"("State(s) in (\"\")"=w354) -> ("States Out"=w353:string)  [unwired: 14 in]
      }
      frame Default {
        w364 = 42 items=["No error", "Argument error", "Memory is full", "Out of zone", "End of file", "File already open", "Generic file I/O error", "File not found", "File permission error", "Disk is full", "Duplicate path", "Too many files open", "System feature not enabled", "Resource file not found", "Cannot add resource", "Resource not found", "Image not found", "Image memory error", "Pen does not exist", "Config type invalid", "Config token not found", "Config parse error", "Config memory error", "Bad external code format", "Bad external code offset", "External code not present", "Null window", "Destroy window error", "Null menu", "Print aborted", "Bad print record", "Print driver error", "Windows error during printing", "Memory error during printing", "Print dialog error", "Generic print error", "Invalid device refnum", "Device not found", "Device parameter error", "Device unit error", "Cannot open device", "Device call aborted", "Generic error", "Cancelled by user", "Object ID too low", "Object ID too high", "Object not in heap", "Unknown heap", "Unknown object (invalid DefProc)", "Unknown object (DefProc not in table)", "Message out of range", "Invalid (null) method", "Unknown message", "Manager call not supported", "Bad address", "Network operation in progress", "Network operation timed out", "Connection is busy", "Network attribute not supported", "Network error", "Address in use", "System out of memory", "Connection aborted", "Connection refused", "Not connected", "Already connected", "Connection closed", "Initialization error (interapplication manager)", "Bad occurrence", "Wait on unbound occurrence handler", "Occurrence queue overflow", "Datalog type conflict", "Unused", "Unrecognized type (interapplication manager)", "Memory corrupt", "Failed to make temporary DLL", "Old CIN version", "Drag socket not found", "Failed to load drop-object", "Failed to register OLE object", "Failed to release OLE object", "Format specifier type mismatch", "Unknown format specifier", "Too few format specifiers", "Too many format specifiers", "Scan failed", "Newer CIN version", "Error converting to variant", "Runtime menu error", "Password tampered", "Variant attribute not found", "Incompatible variant data type", "Event data is not available", "Event Store is not present", "Occurrence is not found", "Event Queue is not created", "Event info is not available", "Refnum passed is NULL", "Error retrieving Class GUID", "Error retrieving CoClass GUID", "Error retrieving TypeLib GUID.", "Bad built application magic bytes.", "Specific driver is different from the specific driver associated with the Logical Name.", "There is no session opened to the class driver.", "Max Error", "MAX - Error with config objects", "MAX - Error loading configuration", "MAX - Group not supported"]
        # "Current State"
        # "Do not delete, rename, or modify this frame.\n(this is used to capture unhandled states and typos)"
        # "Handle mistyped state name (developer tool)"
        n165 = Format Into String(format string="Software Exception: Unhandled State \"%s\"." ("message"), error in=w360, w355) -> (resulting string=w363:string, error out=w362:errorcluster)  [unwired: 1 in]
        n166 = call <vilib>:"Error Cluster From Error Code.vi"("show call chain? (False)"=TRUE, "error in (no error)"=w362, "error message (\"\")"=w363, "error code (0)"=w364) -> ("error out"=w361:errorcluster)  [unwired: 5 in]
        n167 = call <vilib>:"Add State(s) to Queue__jki_lib_state_machine.vi"("State(s) in (\"\")"=w359) -> ("States Out"=w358:string)  [unwired: 14 in]
      }
      frame "Initialize Core Data" {
        # "Do not delete, rename, or modify this frame.\n(this is used to determine panel behavior on exit)"
        # "originally closed?"
        # "exe?"
        # "If panel starts closed or is an EXE, then close it when we exit"
        n168 = property class="VI"() -> ("Front Panel.Open"=w373:bool)  [unwired: 2 in, 2 out]
        n169 = property class="App"() -> ("App.Kind"=w372:T9)  [unwired: 2 in, 2 out]
        n170 = control-ref of="Current VI Reference"() -> (w366:refnum<vi>)
        n171 = Not(x=w373) -> (.not. x?=w370:bool)
        n172 = Equal?(x=w372, y=T9."Run Time System" ("Application:Kind")) -> (x = y?=w369:bool)
        n173 = Or(x=w370, y=w369) -> (x .or. y?=w367:bool)
        n174 = Bundle By Name(cluster=w368, "Core.Current VI Reference"=w366, "Core.Close Panel on Exit?"=w367) -> (w375:T13)
        n175 = call <vilib>:"Add State(s) to Queue__jki_lib_state_machine.vi"("State(s) in (\"\")"=w377) -> ("States Out"=w376:string)  [unwired: 14 in]
      }
      frame "Error Handler" {
        # "Unhandled Error -- Display it"
        # "Handle any errors here.\nYou can also output any states to clean-up after errors occur"
        # "Clear error"
        n176 = call <vilib>:"General Error Handler.vi"("error in (no error)"=w379) -> ()  [unwired: 10 in, 5 out]
        n177 = call <vilib>:"Add State(s) to Queue__jki_lib_state_machine.vi"("State(s) in Front (\"\")"="/* Post Error States", "State(s) in (\"\")"=w383) -> ("States Out"=w382:string)  [unwired: 13 in]
      }
      frame "Exit" {
        # "Do not put any code in this frame.\n(No errors that occur here will be handled.)"
        n178 = call <vilib>:"Add State(s) to Queue__jki_lib_state_machine.vi"("State(s) in (\"\")"=w388) -> ("States Out"=w387:string)  [unwired: 14 in]
      }
      frame "---------- Data ----------" {
        # "Do not put any code in this frame.\n(It is a separator no-op. You can make a copy of this frame to create a new Data frame)"
        n179 = call <vilib>:"Add State(s) to Queue__jki_lib_state_machine.vi"("State(s) in (\"\")"=w392) -> ("States Out"=w391:string)  [unwired: 14 in]
      }
      frame "Data: Initialize" {
        w393 = FALSE  # Fire Continues Allowed
        w395 = u32 0  # Tik1
        w394 = u32 0  # Tik2
        w396 = FALSE  # Jet trigger
        w397 = 0.0  # Discharge timing offset
        w398 = 0.0  # Heater timing offset
        w399 = T14 {"Current VI Reference"=refnum, "Close Panel on Exit?"=FALSE}  # Core
        # "Data names and types of shift register data are defined by this bundle."
        # "Initialize the shift-register data, here.\n(data names are defined by what you wire into the bundle function)"
        n180 = Bundle("Core"=w399, "Heater timing offset"=w398, "Discharge timing offset"=w397, "Jet trigger"=w396, "Tik1"=w395, "Tik2"=w394, "Fire Continues Allowed"=w393) -> (w401:T13)  [unwired: 1 in]
        n181 = call <vilib>:"Add State(s) to Queue__jki_lib_state_machine.vi"("State(s) in (\"\")"=w403) -> ("States Out"=w402:string)  [unwired: 14 in]
      }
      frame "Data: Cleanup" {
        # "Cleanup any data and references, here.\n(this is called automatically, by the Macro: Exit)"
        n182 = Unbundle By Name(w404) -> ("Core.Current VI Reference"=w407:refnum<vi>)
        n183 = Close Reference(reference=w407, error in (no error)=w406) -> (error out=w405:errorcluster)
        n184 = call <vilib>:"Add State(s) to Queue__jki_lib_state_machine.vi"("State(s) in (\"\")"=w409) -> ("States Out"=w408:string)  [unwired: 14 in]
      }
      frame "---------- UI ----------" {
        # "Do not put any code in this frame.\n(It is a separator no-op. You can make a copy of this frame to create a new UI frame)"
        n185 = call <vilib>:"Add State(s) to Queue__jki_lib_state_machine.vi"("State(s) in (\"\")"=w413) -> ("States Out"=w412:string)  [unwired: 14 in]
      }
      frame "UI: Initialize" {
        # "Initialize the User Interface, here.\n(this is called automatically, by the Macro: Init)"
        n186 = call <userlib>:"Fit VI window to Largest Dec__ogtk.vi"() -> ()  [unwired: 6 in, 2 out]
        n187 = call <vilib>:"Add State(s) to Queue__jki_lib_state_machine.vi"("State(s) in (\"\")"=w417) -> ("States Out"=w416:string)  [unwired: 14 in]
      }
      frame "UI: Cursor Set" {
        # "Argument"
        # "Set and Unset Cursor Busy.\n(Usage: \"UI: Cursor Set >> Busy|Idle\")"
        n188 = case shown="\"Idle\", Default" w418 {
          tunnel: w420 -> [w425 w427]
          tunnel: [w424 w426] -> w419
          frame "Idle", Default {
            n189 = call <vilib>:"Unset Busy.vi"("error in (no error)"=w425) -> ("error out"=w424:errorcluster)  [unwired: 10 in]
          }
          frame "Busy" {
            n190 = call <vilib>:"Set Busy.vi"("error in (no error)"=w427) -> ("error out"=w426:errorcluster)  [unwired: 9 in, 1 out]
          }
        }
        n191 = call <vilib>:"Add State(s) to Queue__jki_lib_state_machine.vi"("State(s) in (\"\")"=w423) -> ("States Out"=w422:string)  [unwired: 14 in]
      }
      frame "UI: Front Panel State" {
        # "Argument"
        # "Set Front Panel Open or Closed\n(Usage: \"UI: Front Panel State >> Open|Close\")"
        n192 = Unbundle By Name(w430) -> ("Core.Current VI Reference"=w429:refnum<vi>)
        n193 = case shown="\"Close\"" w428 {
          tunnel: w432 -> [w438 w451]
          tunnel: [w440 w452] -> w431
          tunnel: w429 -> [w439 w449]
          frame "Open", Default {
            n194 = property class="VI"(reference=w439, error in=w438) -> (reference out=w436:refnum<vi>, error out=w437:errorcluster, "Front Panel.Open"=w435:bool)
            n195 = case shown="False" w435 {
              tunnel: [w443 w446] -> w440
              tunnel: w437 -> [w442 w446]
              tunnel: w436 -> [w441 _]
              frame False {
                n196 = invoke class="VI" method="FP.Open"(reference=w441, error in=w442, "Activate"=TRUE, "State"=T10."Standard") -> (error out=w443:errorcluster)  [unwired: 1 in, 4 out]
              }
              frame True {
              }
            }
          }
          frame "Close" {
            n197 = property class="VI"(reference=w449, error in=w451) -> (reference out=w448:refnum<vi>, error out=w450:errorcluster, "Front Panel.Open"=w447:bool)
            n198 = case shown="True" w447 {
              tunnel: [w453 w456] -> w452
              tunnel: w450 -> [w453 w455]
              tunnel: w448 -> [_ w454]
              frame False {
              }
              frame True {
                n199 = invoke class="VI" method="FP.Close"(reference=w454, error in=w455) -> (error out=w456:errorcluster)  [unwired: 1 in, 2 out]
              }
            }
          }
        }
        n200 = call <vilib>:"Add State(s) to Queue__jki_lib_state_machine.vi"("State(s) in (\"\")"=w434) -> ("States Out"=w433:string)  [unwired: 14 in]
      }
      frame "---------- Macro ----------" {
        # "Do not put any code in this frame.\n(It is a separator no-op. You can make a copy of this frame to create a new Macro frame)"
        n201 = call <vilib>:"Add State(s) to Queue__jki_lib_state_machine.vi"("State(s) in (\"\")"=w460) -> ("States Out"=w459:string)  [unwired: 14 in]
      }
      frame "Macro: Initialize" {
        w461 = "Data: Initialize\nInitialize Core Data\nUI: Initialize\nUI: Front Panel State >> Open\nCheck if Fire continues allowed\nInitilize Fire Continues\nInit:MegattenuatorStage"  # Data: Initialize Initialize Core Data UI: Initialize UI: Front Panel State >> Open Check if Fire continues allowed Initilize Fire Continues Init:MegattenuatorStage
        # "Initialization Macro\n(This is called once, when the VI starts)"
        n202 = call <vilib>:"Add State(s) to Queue__jki_lib_state_machine.vi"("State(s) in Front (\"\")"=w461, "State(s) in (\"\")"=w465) -> ("States Out"=w464:string)  [unwired: 13 in]
      }
      frame "Macro: Exit" {
        # "Exit Macro\n(This is called once, when the VI exits)"
        n203 = Unbundle By Name(w475) -> ("Core.Close Panel on Exit?"=w474:bool)
        n204 = Release Queue(queue=w467, force destroy? (F)=TRUE) -> (error out=w466:errorcluster)  [unwired: 1 in, 2 out]
        n205 = call <vilib>:"Clear Errors.vi"("error in (no error)"=w466) -> ()  [unwired: 5 in, 2 out]
        n206 = Select(t="UI: Front Panel State >> Close", s=w474, f="") -> (s? t:f=w471:string)
        n207 = call <vilib>:"Add State(s) to Queue__jki_lib_state_machine.vi"("State(s) in (\"\")"=w471, "State(s) at Back (\"\")"="Data: Cleanup\nExit") -> ("States Out"=w469:string)  [unwired: 13 in]
        n208 = call <vilib>:"Add State(s) to Queue__jki_lib_state_machine.vi"("State(s) in Front (\"\")"=w469, "State(s) in (\"\")"=w478) -> ("States Out"=w477:string)  [unwired: 13 in]
      }
      frame "---------- New Category ----------" {
        # "Template Separator\n(You can make a copy of, or modify, this frame)"
        n209 = call <vilib>:"Add State(s) to Queue__jki_lib_state_machine.vi"("State(s) in (\"\")"=w482) -> ("States Out"=w481:string)  [unwired: 14 in]
      }
      frame "Check Megattenuator Stage Status" {
        n210 = property on="Position.Ch1::44" class="DigNum (strict)"() -> ("Value"=w483:dbl)  [unwired: 2 in, 2 out]
        n211 = case shown="0, 1" w483 {
          tunnel: ["IN" "Unknown/Moving" "OUT"] -> w484
          frame 0, 1 {
            n212 = property on="MoveStage" class="Bool (strict)"("Value"=TRUE) -> ()  [unwired: 2 in, 2 out]
          }
          frame 2, Default {
          }
          frame 149..151 {
            n213 = property on="MoveStage" class="Bool (strict)"("Value"=FALSE) -> ()  [unwired: 2 in, 2 out]
          }
        }
        n214 = property on="CurrentStatus" class="Str"("Value"=w484) -> ()  [unwired: 2 in, 2 out]
        n215 = call <vilib>:"Add State(s) to Queue__jki_lib_state_machine.vi"("State(s) in (\"\")"=w488) -> ("States Out"=w487:string)  [unwired: 14 in]
      }
      frame "Init:MegattenuatorStage" {
        # "Template Separator\n(You can make a copy of, or modify, this frame)"
        n216 = disable-structure shown="Disabled" {
          frame Disabled {
            n217 = flat-sequence {
              frame #0 {
                n218 = call <vilib>:"Set Busy.vi"("disable click? (T)"=TRUE, "cursor ID"=refnum<k1> refnum) -> ()  [unwired: 8 in, 2 out]
              }
              frame #1 {
                n219 = while {
                  tunnel: [w509] -> w501
                  i -> [w504]
                  stop <- w505 stop-if-true
                  n220 = property on="Position.Ch1::44" class="DigNum (strict)"() -> ("Value"=w509:dbl)  [unwired: 2 in, 2 out]
                  n221 = Equal?(x=50, y=w504) -> (x = y?=w502:bool)
                  n222 = Not Equal?(x=w509, y=0.0) -> (x != y?=w506:bool)
                  n223 = Wait (ms)(milliseconds to wait=u32 100) -> ()  [unwired: 1 out]
                  n224 = Or(x=w506, y=w502) -> (x .or. y?=w505:bool)
                }
                n225 = case shown="0, 1" w501 {
                  tunnel: ["IN" "Unknown" "OUT"] -> w500
                  frame 0, 1 {
                    n226 = property on="MoveStage" class="Bool (strict)"("Value"=TRUE) -> ()  [unwired: 2 in, 2 out]
                  }
                  frame 2, Default {
                    n227 = property on="MoveStage" class="Bool (strict)"("DisabledEnum"=T8."Disabled" ("Disabled")) -> ()  [unwired: 2 in, 2 out]
                  }
                  frame 149..151 {
                    n228 = property on="MoveStage" class="Bool (strict)"("Value"=FALSE) -> ()  [unwired: 2 in, 2 out]
                  }
                }
                n229 = property on="CurrentStatus" class="Str"("Value"=w500) -> ()  [unwired: 2 in, 2 out]
              }
              frame #2 {
                n230 = call <vilib>:"Unset Busy.vi"() -> ()  [unwired: 11 in, 1 out]
              }
            }
          }
          frame Enabled {
          }
        }
        n231 = call <vilib>:"Add State(s) to Queue__jki_lib_state_machine.vi"("State(s) in (\"\")"=w497) -> ("States Out"=w496:string)  [unwired: 14 in]
      }
      frame "CheckTimeFire" {
        # "Your code here.\n(You can make a copy of, or modify, this frame)"
        n232 = Unbundle By Name(w522) -> ("Tik1"=w527:u32)
        n233 = Tick Count (ms)() -> (millisecond timer value=w529:u32)
        n234 = Unbundle By Name(w522) -> ("Fire Continues Allowed"=w519:bool)
        n235 = Reciprocal(x="Rate (Hz)") -> (1/x=w518:dbl)
        n236 = Subtract(x=w529, y=w527) -> (x-y=w530:u32)
        n237 = Multiply(x=1000.0, y=w518) -> (x*y=w517:dbl)
        n238 = Greater?(x=w530, y=w517) -> (0:w525:bool)
        n239 = And(x=w525, y="value0::22") -> (x .and. y?=w521:bool)
        n240 = And(x=w519, y=w521) -> (x .and. y?=w520:bool)
        n241 = case shown="True" w520 {
          tunnel: w529 -> [_ w537]
          tunnel: [w535 w537] -> w528
          tunnel: w527 -> [w535 _]
          tunnel: [_ "Action: Fire" ("State(s) in Front (\"\")")] -> w524
          frame False {
          }
          frame True {
          }
        }
        n242 = Bundle By Name(cluster=w522, "Tik1"=w528) -> (w531:T13)
        n243 = call <vilib>:"Add State(s) to Queue__jki_lib_state_machine.vi"("State(s) in Front (\"\")"=w524, "State(s) in (\"\")"=w534) -> ("States Out"=w533:string)  [unwired: 13 in]
        "Fire continues Indicator" <- "value0::22"
      }
      frame "Initilize Fire Continues" {
        # "Your code here.\n(You can make a copy of, or modify, this frame)"
        n244 = Unbundle By Name(w541) -> ("Fire Continues Allowed"=w540:bool)
        n245 = property on="value0::22" class="Bool (strict)"(error in=w543, "Visible"=w540) -> (error out=w542:errorcluster)  [unwired: 1 in, 1 out]
        n246 = Not(x=w540) -> (.not. x?=w538:bool)
        n247 = property on="Fire continues Indicator" class="Bool (strict)"(error in=w542, "Visible"=w538) -> (error out=w539:errorcluster)  [unwired: 1 in, 1 out]
        n248 = call <vilib>:"Add State(s) to Queue__jki_lib_state_machine.vi"("State(s) in (\"\")"=w545) -> ("States Out"=w544:string)  [unwired: 14 in]
      }
      frame "Check if Fire continues allowed" {
        # "Check if it is allowed computer"
        # "Your code here.\n(You can make a copy of, or modify, this frame)"
        n249 = String To IP() -> (0:w553:u32)  [unwired: 1 in]
        n250 = IP To String(1:TRUE ("dot notation? (F)"), 2:w553) -> (0:w554:string)
        n251 = Equal?(x=w554, y="192.168.14.2") -> (x = y?=w548:bool)
        n252 = Not(x=w548) -> (.not. x?=w549:bool)
        n253 = Bundle By Name(cluster=w551, "Fire Continues Allowed"=w548) -> (w550:T13)
        n254 = property on="Allow Fire Continues" class="Bool (strict)"(error in=w547, "Visible"=w549) -> (error out=w546:errorcluster)  [unwired: 1 in, 1 out]
        n255 = call <vilib>:"Add State(s) to Queue__jki_lib_state_machine.vi"("State(s) in (\"\")"=w557) -> ("States Out"=w556:string)  [unwired: 14 in]
      }
      frame "CheckTime2" {
        # "Your code here.\n(You can make a copy of, or modify, this frame)"
        n256 = Unbundle By Name(w566) -> ("Tik2"=w559:u32)
        n257 = Tick Count (ms)() -> (millisecond timer value=w561:u32)
        n258 = Subtract(x=w561, y=w559) -> (x-y=w564:u32)
        n259 = Greater?(x=w564, y=5000) -> (0:w562:bool)
        n260 = case shown="True" w562 {
          tunnel: w561 -> [_ w572]
          tunnel: [w570 w572] -> w560
          tunnel: w559 -> [w570 _]
          tunnel: [_ "Action: update expt vars\nAction: save screenshot"] -> w558
          frame False {
          }
          frame True {
          }
        }
        n261 = Bundle By Name(cluster=w566, "Tik2"=w560) -> (w565:T13)
        n262 = call <vilib>:"Add State(s) to Queue__jki_lib_state_machine.vi"("State(s) in Front (\"\")"=w558, "State(s) in (\"\")"=w569) -> ("States Out"=w568:string)  [unwired: 13 in]
      }
      frame "Action: Fire" {
        n263 = property on="fire::10" class="Str"(error in=w574, "Val(Sgnl)"="fire>>force" ("Value (Signaling)")) -> (error out=w573:errorcluster)  [unwired: 1 in, 1 out]
        n264 = call <vilib>:"Add State(s) to Queue__jki_lib_state_machine.vi"("State(s) in (\"\")"=w578) -> ("States Out"=w577:string)  [unwired: 14 in]
      }
      frame "Action: update expt vars" {
        # "Your code here.\n(You can make a copy of, or modify, this frame)"
        n265 = call <vilib>:"Add State(s) to Queue__jki_lib_state_machine.vi"("State(s) in (\"\")"=w582) -> ("States Out"=w581:string)  [unwired: 14 in]
      }
      frame "Action: SendScanParameters" {
        # "Your code here.\n(You can make a copy of, or modify, this frame)"
        n266 = Bundle("value4::42"="value4::42", "B") -> (w593:cluster{"value4::42":dbl, string})  [unwired: 1 in]
        n267 = Bundle("value8::42"="value8::42", "D") -> (w590:cluster{"value8::42":dbl, string})  [unwired: 1 in]
        n268 = Bundle("value9::42"="value9::42", "F") -> (w585:cluster{"value9::42":dbl, string})  [unwired: 1 in]
        n269 = Bundle("value10::42"="value10::42", "H") -> (w584:cluster{"value10::42":dbl, string})  [unwired: 1 in]
        n270 = Build Array(w593, w590, w585, w584) -> (w583:cluster{"value10::42":dbl, string}[])
        "Jet On Times" <- w583
        n271 = call "BELLA PW scan mode shot control shutter.vi"("PostScanRate"="value6::42", "ScanShotControl"="value0::43") -> ("error out"=w600:errorcluster, "delay D to set"=w596:dbl)  [unwired: 8 in]
        n272 = property on="Delay.Ch D::10" class="DigNum (strict)"("Val(Sgnl)"=w596) -> ()  [unwired: 2 in, 2 out]
        n273 = call "Jet in scan on or off.vi"("error in (no error)"=w600, "Jet On Times"=w583, "GasJetOn"="value1::43") -> ("error out"=w598:errorcluster)  [unwired: 8 in]
        n274 = flat-sequence {
          tunnel: w598 -> [_]
          frame #0 {
            n275 = call "TimeoutDialog.vi"("message 2"="expt editor set up" ("message"), "Timeout(ms)"=u32 1000) -> ()  [unwired: 9 in]
          }
        }
        n276 = call <vilib>:"Add State(s) to Queue__jki_lib_state_machine.vi"("State(s) in (\"\")"=w605) -> ("States Out"=w604:string)  [unwired: 14 in]
      }
      frame "Action: save screenshot" {
        # "Your code here.\n(You can make a copy of, or modify, this frame)"
        n277 = case shown="True" "Save \ncreenshots" {
          frame False {
          }
          frame True {
            n278 = invoke class="VI" method="FP.Get Image"() -> ("image data"=w615:T11)  [unwired: 6 in, 5 out]
            n279 = call <vilib>:"Write PNG File.vi"("image data"=w615, "path to PNG file"=path "N:/data/ECS dumps/Logmaker Screenshot/frontpanel.png" ("report file path")) -> ("error out"=→"error out":errorcluster)  [unwired: 8 in, 1 out]
          }
        }
        n280 = call <vilib>:"Add State(s) to Queue__jki_lib_state_machine.vi"("State(s) in (\"\")"=w612) -> ("States Out"=w611:string)  [unwired: 14 in]
      }
    }
  }
  n281 = for {
    N: 25 -> [_]
    tunnel: w4 -> [w618]
    tunnel: [w618] -> w3
    tunnel: [w616] -> w1
    stop <- w616 stop-if-true
    n282 = local read "got manpar ofi data"() -> (w620:bool)
    n283 = local read "got manpar ofi bool data"() -> (w619:bool)
    n284 = Wait (ms)(milliseconds to wait=u32 1000) -> ()  [unwired: 1 out]
    n285 = And(x=w620, y=w619) -> (x .and. y?=w616:bool)
  }
  n286 = disable-structure shown="Disabled" {
    frame Disabled {
    }
    frame Enabled {
    }
  }
  n287 = case shown="True" w1 {
    tunnel: w3 -> [_ w621]
    frame False {
    }
    frame True {
      n288 = call <userlib>:"Wait (ms)__ogtk.vi"("error in (no error)"=w621, "milliseconds to wait"=u32 3000) -> ("error out"=w623:errorcluster)  [unwired: 8 in, 1 out]
      n289 = property on="set expt editor" class="Bool (strict)"(error in=w623, "Val(Sgnl)"=TRUE ("Value (Signaling)")) -> ()  [unwired: 1 in, 2 out]
    }
  }
  n290 = disable-structure shown="Disabled" {
    frame Disabled {
    }
    frame Enabled {
    }
  }
  "CurrentStatus" <- ""
